vi "44 Config File Read Telecoms (x64-2018).vi"() -> (0 "Port":i32, 1 "IP":string, 2 "ID":string)   [LabVIEW 2017]
uses:
  <vilib>/Utility/config.llb/Read Key (String).vi
  <vilib>/Utility/config.llb/Read Key (I32).vi
  <vilib>/Utility/config.llb/NI_LVConfig.lvlib
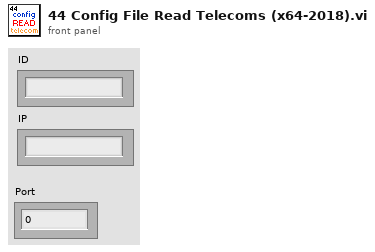
[diagram p1: front panel]
types:
  T1 = typedef "NI_LVConfig.lvlib/Config Data RefNum.ctl" = refnum<k1>
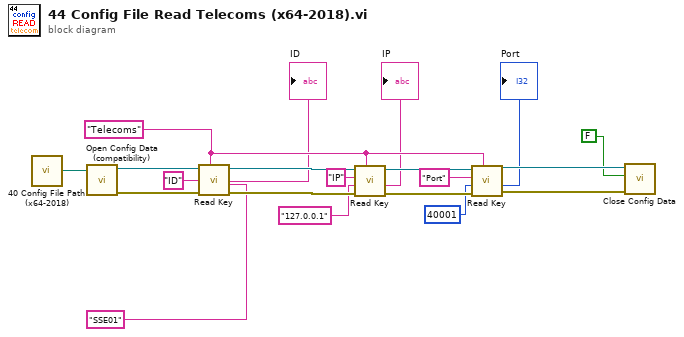
[diagram p0: block diagram]
diagram:
  w11 = "Telecoms" ("section")
  n1 = call "40 Config File Path (x64-2018).vi"() -> ("Configuration File Path"=w1:path)
  n2 = call <vilib>:"Open Config Data (compatibility).vi"("configuration file path"=w1) -> ("error out"=w19:errorcluster, "refnum"=w20:T1)  [unwired: 8 in, 1 out]
  n3 = call-poly <vilib>:"Read Key.vi"("section"=w11, "error in (no error)"=w19, "default value"="SSE01" ("key"), "key"="ID", "refnum"=w20) -> ("error out"=w15:errorcluster, "value"=→"ID":string, "refnum out"=w17:T1)  [unwired: 3 in, 1 out]
  n4 = call-poly <vilib>:"Read Key.vi"("section"=w11, "error in (no error)"=w15, "default value"="127.0.0.1" ("key"), "key"="IP", "refnum"=w17) -> ("error out"=w13:errorcluster, "value"=→"IP":string, "refnum out"=w14:T1)  [unwired: 3 in, 1 out]
  n5 = call-poly <vilib>:"Read Key.vi"("section"=w11, "error in (no error)"=w13, "default value"=40001, "key"="Port", "refnum"=w14) -> ("error out"=w5:errorcluster, "value"=→"Port":i32, "refnum out"=w6:T1)  [unwired: 3 in, 1 out]
  n6 = call <vilib>:"Close Config Data.vi"("error in (no error)"=w5, "write file if changed (T)"=FALSE ("write configuration file? (T)"), "refnum"=w6) -> ()  [unwired: 7 in, 2 out]
